vi "Convert to AI with Conversion Time Module.vi"(8 "error in":errorcluster, 9 "9224 in":refnum<class "9224.lvclass">, 10 "slot ref in":T1 format="%.0x", 11 "module in":refnum<class "Module.lvclass">) -> (0 "error out":errorcluster, 2 "slot ref out":T1 format="%.0x", 3 "module out":refnum<class "Module.lvclass">)   [LabVIEW 2017, in "Scan Engine Scripting.lvlib"]
uses:
  Scan Engine Scripting.lvlib
  Modules/Module/Module.lvclass
  <vilib>/NI Veristand/Custom Device API/Custom Device Item Ref.ctl
  Modules.lvlibp/9224/9224.lvclass
  Modules/Mode Classes/Analog Inputs with Conversion Time Mode/Analog Input with Conversion Time Mode.lvclass
  C:/Users/nitest/Documents/niveristand-scan-engine-ethercat-custom-device/Custom Device Source/Scripting/Modules/Mode Classes/Mode/Mode.lvclass
  8298e5b1-cf4c-42d6-8d85-14c36b5a5072.vi
  <vilib>/NI Veristand/Custom Device API/Custom Device API.lvlib
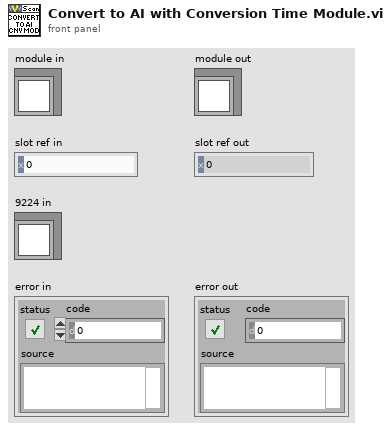
[diagram p1: front panel]
types:
  T1 = typedef "Custom Device API.lvlib/Custom Device Item Ref.ctl" = u64
  T2 = typedef "Modules.lvlibp/9224.lvclass/Conversion Time.ctl" = u16
  T3 = typedef "Scan Engine Scripting.lvlib/analog channel settings.ctl" = cluster{"name":string, "default value":dbl}
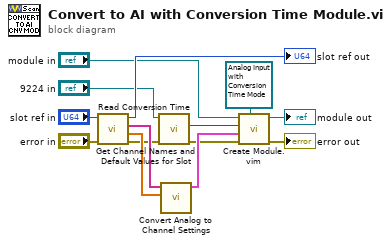
[diagram p0: block diagram]
diagram:
  n1 = call "Get Channel Names and Default Values for Slot.vi"("error in"="error in", "slot ref in"="slot ref in") -> ("error out"=w9:errorcluster, "channel default values"=w10:dbl[], "channel names"=w11:string[], "slot ref out"=→"slot ref out":T1)  [unwired: 6 in]
  n2 = call-dynamic "Read Conversion Time.vi"("error in"=w9, "9224 in"="9224 in") -> ("error out"=w5:errorcluster, "Conversion Time"=w7:T2)  [unwired: 7 in, 1 out]
  n3 = call "Convert Analog to Channel Settings.vi"("channel default values"=w10, "channel names"=w11) -> ("channel settings"=w6:T3[])  [unwired: 9 in]
  n4 = call "Create Module.vim"("mode in"=refnum<class "Analog Input with Conversion Time Mode.lvclass"> refnum ("Scan Engine Scripting.lvlib:Analog Input with Conversion Time Mode.lvclass"), "error in"=w5, "channel settings"=w6, "mode settings"=w7, "module in"="module in") -> ("error out"=→"error out":errorcluster, "module out"=→"module out":refnum<class "Module.lvclass">)  [unwired: 5 in]
